vi "Get System Asset.vi"() -> (3 "asset":T1)   [LabVIEW 2023, in "Logger.lvclass"]
uses:
  Logger.lvclass
  <resource>/objmgr/nisysapi.rc
  <vilib>/nisyscfg/nisyscfg.lvlib
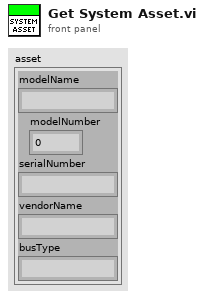
[diagram p1: front panel]
types:
  T1 = cluster{"modelName":string, "modelNumber":i32, "serialNumber":string, "vendorName":string, "busType":string}
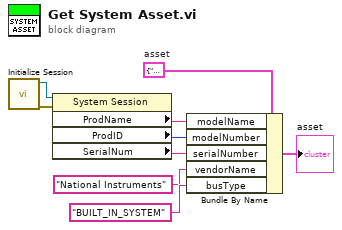
[diagram p0: block diagram]
diagram:
  w8 = T1 {"modelName"="", "modelNumber"=0, "serialNumber"="", "vendorName"="", "busType"="BUILT_IN_SYSTEM"}  # asset
  n1 = call <vilib>:"Initialize Session.vi"() -> ("error out"=w5:errorcluster, "Session out"=w6:refnum<k21>)  [unwired: 10 in]
  n2 = property class="System Session"(reference=w6, error in=w5) -> ("ProdName"=w4:string, "ProdID"=w3:i32, "SerialNum"=w2:string)  [unwired: 2 out]
  n3 = Bundle By Name(cluster=w8, "modelName"=w4, "modelNumber"=w3, "serialNumber"=w2, "vendorName"="National Instruments", "busType"="BUILT_IN_SYSTEM") -> (→"asset":T1)
